vi "SensorDataGlobal.vi"() -> ()   [LabVIEW 2017]
panel:
  in  "Robot Lift Data":T1
  in  "Drive Data":T2
  in  "Cube Lift Position":i32
  in  "Re-Zero Gyro?":bool
  in  "Gyro Data":cluster{"Heading":dbl, "Gyro Raw":dbl}
  out "Intake Switch":bool
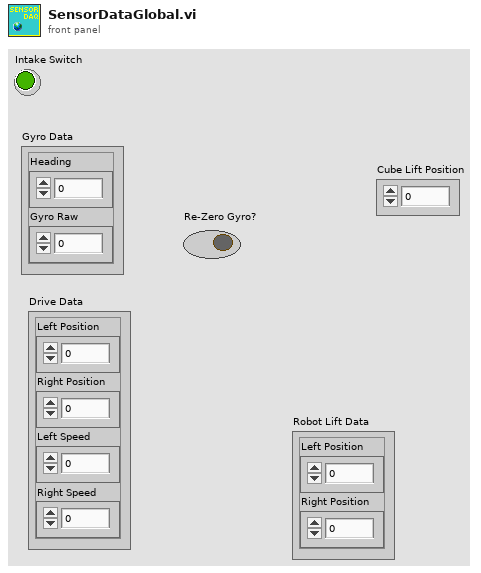
[diagram p1: front panel]
types:
  T1 = cluster{"Left Position":i32, "Right Position":i32}
  T2 = cluster{"Left Position":i32, "Right Position":i32, "Left Speed":i32, "Right Speed":i32}
diagram:
